vi "VI-Create Reg XControl Events.vi"(0 "VI ref in":refnum<vi>, 2 "application refnum":refnum<vi>, 7 "Insert? (T)":bool=TRUE, 11 "error in (no error)":errorcluster) -> (4 "VI ref out":refnum<vi>, 15 "error out":errorcluster)   [LabVIEW 2015]
uses:
  <vilib>/Utility/miscctls.llb/LVPointTypeDef.ctl
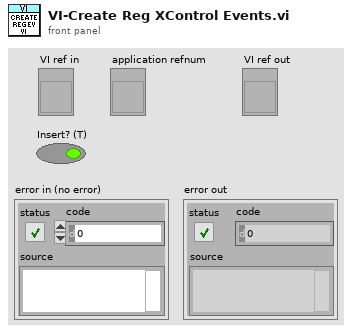
[diagram p1: front panel]
types:
  T1 = typedef "LVPointTypeDef.ctl" = cluster{"Horizontal":i16, "Vertical":i16}
  T2 = typedef "VI-Reg Event Components.ctl" = cluster{"Refs":refnum<vi>, "Dummy":refnum<vi>, "Index Array":refnum<vi>, "bundle":refnum<vi>, "unbundle":refnum<vi>, "reg":refnum<vi>, "invoke":refnum<vi>, "temp":refnum<vi>}
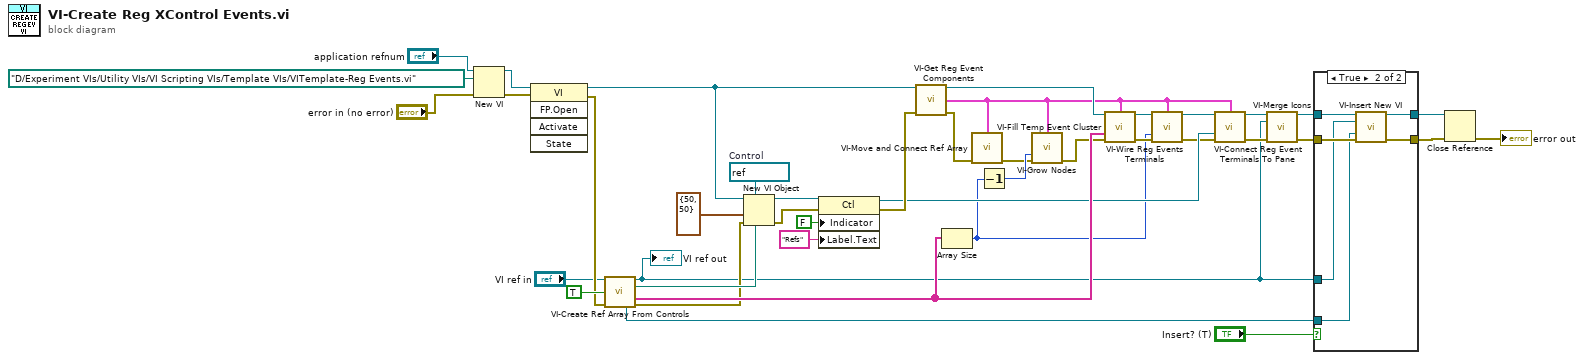
[diagram p0: block diagram]
diagram:
  w35 = refnum<vi> refnum  # Control
  n1 = New VI(8:"error in (no error)", 10:path "D:/Experiment VIs/Utility VIs/VI Scripting VIs/Template VIs/VITemplate-Reg Events.vi" ("template"), 11:"application refnum") -> (0:w40:errorcluster, 3:w41:refnum<vi>)  [unwired: 4 in]
  n2 = invoke class="VI" method="FP.Open"(reference=w41, error in=w40) -> (reference out=w36:refnum<vi>, error out=w27:errorcluster)  [unwired: 3 in, 3 out]
  n3 = call "VI-Create Ref Array From Controls.vi"("VI ref in"="VI ref in", "Create typedef?"=TRUE, "error in (no error)"=w27) -> ("VI ref out"=w1:refnum<vi>, "typedef path"=w38:path, "Names"=w29:string[], "BldArr Refnum"=w20:refnum<vi>, "error out"=w26:errorcluster)  [unwired: 8 in]
  "VI ref out" <- w1
  n4 = New VI Object(vi object class=w35, owner refnum=w36, position/next to=T1 {"Horizontal"=50, "Vertical"=50} ("location"), 6:w38, 8:w26) -> (object refnum=w34:refnum<vi>, 0:w33:errorcluster)  [unwired: 3 in]
  n5 = property class="Ctl"(reference=w34, error in=w33, "Indicator"=FALSE, "Label.Text"="Refs") -> (reference out=w23:refnum<vi>, error out=w37:errorcluster)
  n6 = call "VI-Get Reg Event Components.vi"("VI in"=w36, "error in (no error)"=w37) -> ("VI out"=w14:refnum<vi>, "Components"=w7:T2, "error out"=w17:errorcluster)  [unwired: 10 in, 1 out]
  n7 = Array Size(array=w29) -> (size(s)=w10:i32)
  n8 = call "VI-Move and Connect Ref Array.vi"("Components"=w7, "error in (no error)"=w17) -> ("error out"=w15:errorcluster)  [unwired: 13 in]
  n9 = Decrement(x=w10) -> (x-1=w16:i32)
  n10 = call "VI-Grow Nodes.vi"("Components"=w7, "Numeric"=w16, "error in (no error)"=w15) -> ("error out"=w13:errorcluster)  [unwired: 12 in]
  n11 = call "VI-Fill Temp Event Cluster.vi"("VI in"=w14, "Components"=w7, "Names"=w29, "error in (no error)"=w13) -> ("VI out"=w11:refnum<vi>, "error out"=w12:errorcluster)  [unwired: 10 in]
  n12 = call "VI-Wire Reg Events Terminals.vi"("VI in"=w11, "Components"=w7, "Num refs"=w10, "error in (no error)"=w12) -> ("VI out"=w9:refnum<vi>, "error out"=w8:errorcluster)  [unwired: 10 in]
  n13 = call "VI-Connect Reg Event Terminals To Pane.vi"("VI in"=w9, "Components"=w7, "Ref array"=w23, "error in (no error)"=w8) -> ("VI out"=w4:refnum<vi>, "error out"=w2:errorcluster)  [unwired: 10 in]
  n14 = call "VI-Merge Icons.vi"("VI in"=w4, "VI ref in"=w1, "error in (no error)"=w2) -> ("VI out"=w5:refnum<vi>, "error out"=w3:errorcluster)  [unwired: 11 in]
  n15 = case shown="True" "Insert? (T)" {
    tunnel: w5 -> [w43 w49]
    tunnel: w3 -> [w42 w48]
    tunnel: [w42 w47] -> w22
    tunnel: [w43 w46] -> w21
    tunnel: w20 -> [_ w44]
    tunnel: w1 -> [_ w45]
    frame False {
    }
    frame True {
      n16 = call "VI-Insert New VI.vi"("VI in"=w49, "Insert VI ref"=w45, "BldArr Refnum"=w44, "error in (no error)"=w48) -> ("VI out"=w46:refnum<vi>, "error out"=w47:errorcluster)  [unwired: 10 in]
    }
  }
  n17 = Close Reference(reference=w21, error in (no error)=w22) -> (error out=→"error out":errorcluster)
